vi "Simple Loop Get Images to Host GUI.vi"() -> ()   [LabVIEW 2017]
uses:
  <vilib>/vision/NI_Vision_Development_Module.lvlib
  IMAQCV/IMAQCV.lvlib
  IMAQCV/PIIO.lvlib
panel:
  out "Loop Rate (Hz)":u32
  in  "Image Size":T1(ring)
  in  "Image Index":u32
  in  "color":bool
  in  "Save Image":bool
  in  "Image File Path":path=path "c:/vision/project-01/camera-000.jpg"
  in  "stop":bool
  out "camera image":T2(plugin-control)
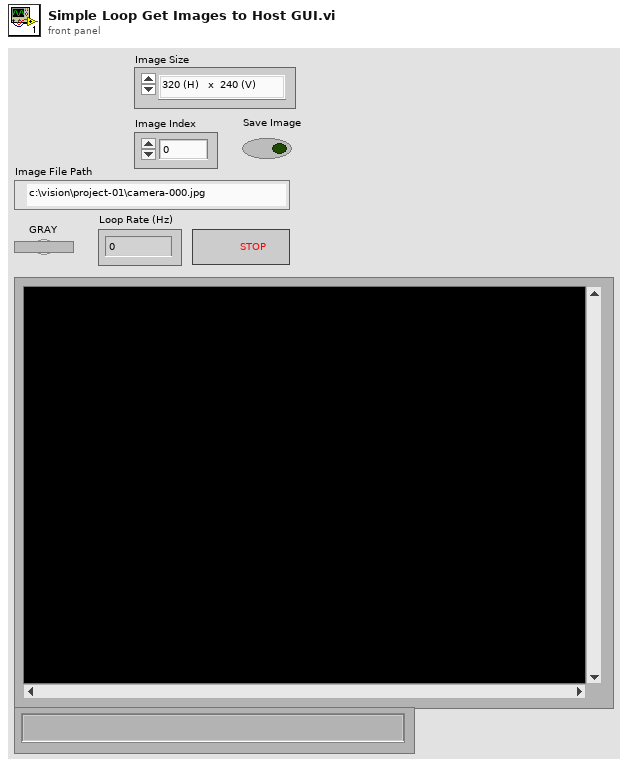
[diagram p1: front panel]
types:
  T1 = enum16{"320 (H)   x  240 (V)", "352(H)    x  288 (V)", "640 (H)   x  480 (V) ", "800 (H)   x  600 (V)", "1024 (H) x  768 (V)", "1280 (H) x  720 (V)", "1280 (H) x  960 (V)", "1280 (H) x 1024 (V)", "1920 (H) x 1080 (V)"}
  T2 = typedef "IMAQ Image.ctl" = refnum<image>
  T3 = typedef "Image Type" = u32
  T4 = typedef "IMAQCV.lvlib/IMAQCV Image.ctl" = refnum<vi>
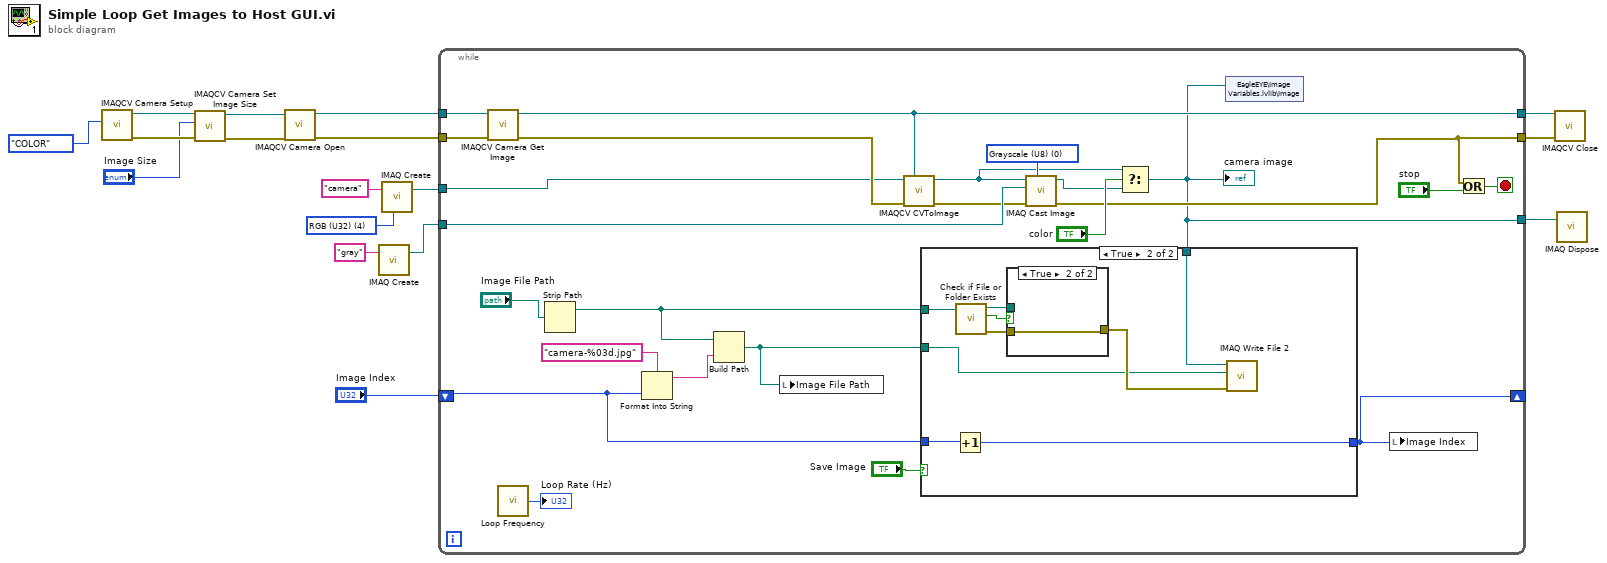
[diagram p0: block diagram]
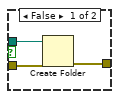
[diagram p3: hidden frame]
diagram:
  w16 = T3 4 items=["Grayscale (U8)", "Grayscale (I16)", "Grayscale (SGL)", "Complex (CSG)", "RGB (U32)", "HSL (U32)", "RGB (U64)", "Grayscale (U16)"] ("Image Type")
  n1 = call "IMAQCV Camera Setup.vi"("type"=enum16{"GRAY", "COLOR"}."COLOR") -> ("error out"=w10:errorcluster, "image out"=w9:T4)  [unwired: 9 in]
  n2 = call "IMAQCV Camera Set Image Size.vi"("error in (no error)"=w10, "Image Size"="Image Size", "image in"=w9) -> ("error out"=w8:errorcluster, "image out"=w7:T4)  [unwired: 7 in]
  n3 = call "IMAQCV Camera Open.vi"("error in (no error)"=w8, "image in"=w7) -> ("error out"=w6:errorcluster, "image out"=w5:T4)  [unwired: 8 in]
  n4 = call "IMAQ Create"("Image Name"="gray") -> ("New Image"=w14:T2)  [unwired: 3 in, 2 out]
  n5 = call "IMAQ Create"("Image Name"="camera", "Image Type"=w16) -> ("New Image"=w17:T2)  [unwired: 2 in, 2 out]
  n6 = while {
    tunnel: w5 -> [w26]
    tunnel: w17 -> [w21]
    tunnel: w14 -> [w38]
    tunnel: [w18] -> w12
    tunnel: [w22] -> w1
    shift-right: [w28] -> _
    shift-left: "Image Index" -> [w29]
    tunnel: w6 -> [w27]
    tunnel: [w20] -> w2
    stop <- w39 stop-if-true
    w41 = T3 0 items=["Grayscale (U8)", "Grayscale (I16)", "Grayscale (SGL)", "Complex (CSG)", "RGB (U32)", "HSL (U32)", "RGB (U64)", "Grayscale (U16)"] ("Image Type")
    n7 = call "IMAQCV Camera Get Image.vi"("error in (no error)"=w27, "image in"=w26) -> ("error out"=w25:errorcluster, "image out"=w22:T4)  [unwired: 8 in]
    n8 = call "Loop Frequency.vi"() -> ("Loop Rate (Hz)"=→"Loop Rate (Hz)":u32)  [unwired: 1 out]
    n9 = Strip Path(path="Image File Path") -> (stripped path=w30:path)  [unwired: 1 out]
    n10 = Format Into String(format string="camera-%03d.jpg", w29) -> (resulting string=w32:string)  [unwired: 2 in, 1 out]
    n11 = Build Path(base path=w30, name or relative path=w32) -> (appended path=w31:path)
    n12 = local write "Image File Path"(w31) -> ()
    n13 = call "IMAQCV CVToImage.vi"("cvimage in"=w22, "error in (no error)"=w25, "Variant In"=w21) -> ("error out"=w24:errorcluster, "Variant Out"=w23:refnum<image>)  [unwired: 7 in]
    n14 = call "IMAQ Cast Image"("Image Type"=w41, "error in (no error)"=w24, "Image Dst"=w38, "Image Src"=w23) -> ("error out"=w20:errorcluster, "Image Dst Out"=w35:T2)  [unwired: 6 in]
    n15 = Select(t=w23, s="color", f=w35) -> (s? t:f=w18:T2)
    "camera image" <- w18
    n16 = case shown="True" "Save Image" {
      tunnel: w18 -> [_ w51]
      tunnel: w31 -> [_ w45]
      tunnel: w30 -> [_ w50]
      tunnel: w29 -> [w42 w44]
      tunnel: [w42 w43] -> w28
      frame False {
      }
      frame True {
        n17 = Increment(x=w44) -> (x+1=w43:u32)
        n18 = call <vilib>:"Check if File or Folder Exists.vi"("path"=w50) -> ("error out"=w47:errorcluster, "file or folder exists?"=w49:bool, "dup path"=w48:path)  [unwired: 8 in]
        n19 = case shown="True" w49 {
          tunnel: w48 -> [w54 _]
          tunnel: w47 -> [w53 w55]
          tunnel: [w52 w55] -> w46
          frame False {
            n20 = Create Folder(path (use dialog)=w54, error in=w53) -> (error out=w52:errorcluster)  [unwired: 1 in, 2 out]
          }
          frame True {
          }
        }
        n21 = call-poly "IMAQ Write File 2"("error in (no error)"=w46, "File Path"=w45, "Image"=w51) -> ()  [unwired: 7 in, 2 out]
      }
    }
    n22 = shared-variable "EagleEYE\\Image Variables.lvlib\\Image"(w18) -> ()  [unwired: 1 in, 1 out]
    n23 = local write "Image Index"(w28) -> ()
    n24 = Or(x=w20, y="stop") -> (x .or. y?=w39:bool)
  }
  n25 = call "IMAQCV Close.vi"("error in (no error)"=w2, "Image"=w1) -> ()  [unwired: 9 in, 1 out]
  n26 = call "IMAQ Dispose"("Image"=w12) -> ()  [unwired: 5 in, 1 out]
